vi "Interpolate Points.vi"(1 "End Point":cluster{"X":dbl, "Y":dbl}, 2 "Distance between Points":dbl, 3 "Start Point":cluster{"X":dbl, "Y":dbl}) -> (0 "Output Point Array":cluster{"X":dbl, "Y":dbl}[](array[cluster]))   [LabVIEW 2013]
doc: "This VI interpolates at specified intervals between two points."
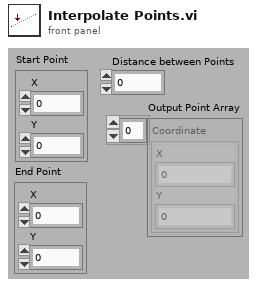
[diagram p1: front panel]
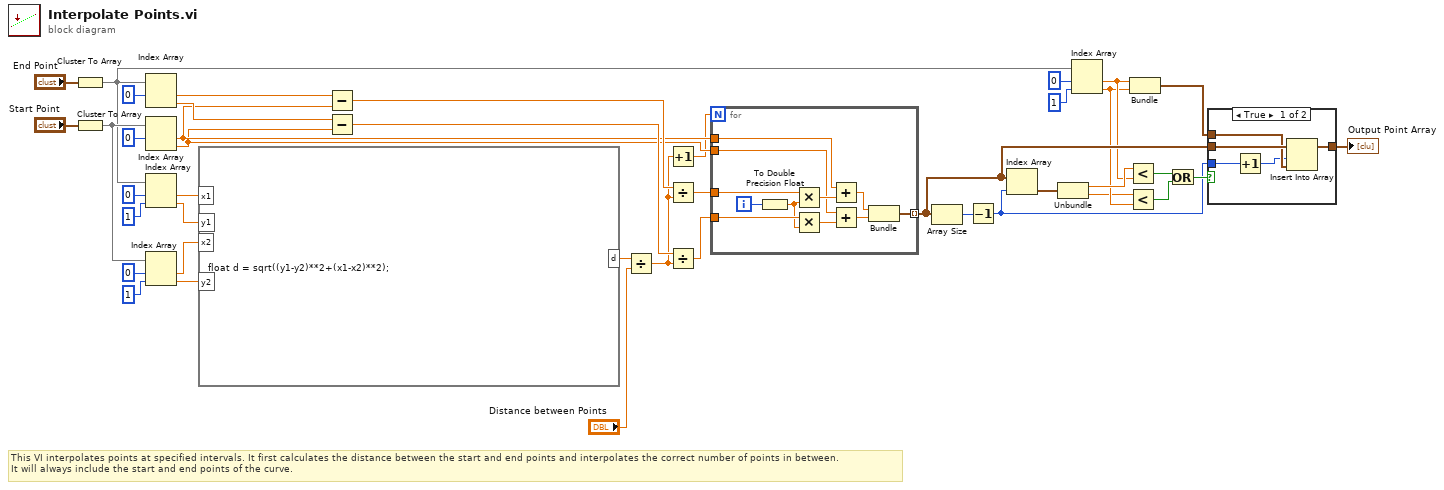
[diagram p0: block diagram]
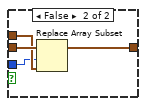
[diagram p2: hidden frame]
diagram:
  # "This VI interpolates points at specified intervals. It first calculates the distance between the start and end points and interpolates the correct number of points in between. \nIt will always include the start and end points of the curve."
  n1 = Cluster To Array(cluster="End Point") -> (array=w13:dbl[])
  n2 = Cluster To Array(cluster="Start Point") -> (array=w14:dbl[])
  n3 = Index Array(array=w13, index #1=0 ("index")) -> (element #1=w39:dbl, element #2=w36:dbl)  [unwired: 1 in]
  n4 = Index Array(array=w14, index #1=0 ("index")) -> (element #1=w35:dbl, element #2=w33:dbl)  [unwired: 1 in]
  n5 = Index Array(array=w13, index #1=0 ("index"), index #2=1 ("index")) -> (element #1=w24:dbl, element #2=w23:dbl)
  n6 = Index Array(array=w14, index #1=0 ("index"), index #2=1 ("index")) -> (element #1=w26:dbl, element #2=w25:dbl)
  n7 = formula code="float d = sqrt((y1-y2)**2+(x1-x2)**2);"("x1"=w24, "y1"=w23, "x2"=w26, "y2"=w25) -> ("d"=w22:dbl)
  n8 = Subtract(x=w39, y=w35) -> (x-y=w38:dbl)
  n9 = Subtract(x=w36, y=w33) -> (x-y=w37:dbl)
  n10 = Divide(x=w22, y="Distance between Points") -> (x/y=w20:dbl)
  n11 = Increment(x=w20) -> (x+1=w31:dbl)
  n12 = Divide(x=w38, y=w20) -> (x/y=w34:dbl)
  n13 = Divide(x=w37, y=w20) -> (x/y=w32:dbl)
  n14 = for {
    N: w31 -> [_]
    tunnel: w35 -> [w52]
    tunnel: w34 -> [w51]
    tunnel: w33 -> [w49]
    tunnel: w32 -> [w48]
    tunnel: [w44] -> w7 mode=indexing
    i -> [w43]
    n15 = To Double Precision Float(number=w43) -> (double precision float=w42:dbl)
    n16 = Multiply(x=w51, y=w42) -> (x*y=w50:dbl)
    n17 = Multiply(x=w48, y=w42) -> (x*y=w47:dbl)
    n18 = Add(x=w52, y=w50) -> (x+y=w46:dbl)
    n19 = Add(x=w49, y=w47) -> (x+y=w45:dbl)
    n20 = Bundle(w46, w45) -> (w44:cluster{dbl, dbl})  [unwired: 1 out]
  }
  n21 = Array Size(array=w7) -> (size(s)=w16:i32)
  n22 = Decrement(x=w16) -> (x-1=w6:i32)
  n23 = Index Array(array=w7, index=w6) -> (element=w5:cluster{dbl, dbl})
  n24 = Unbundle(w5) -> (w4:dbl, w1:dbl)
  n25 = Index Array(array=w13, index #1=0 ("index"), index #2=1 ("index")) -> (element #1=w3:dbl, element #2=w2:dbl)
  n26 = Less?(x=w4, y=w3) -> (x < y?=w9:bool)
  n27 = Less?(x=w1, y=w2) -> (x < y?=w10:bool)
  n28 = Bundle("X"=w3, "X"=w2) -> (w17:cluster{"X":dbl, "X":dbl})  [unwired: 1 in]
  n29 = Or(x=w9, y=w10) -> (x .or. y?=w8:bool)
  n30 = case shown="True" w8 {
    tunnel: w7 -> [w57 w61]
    tunnel: w17 -> [w56 w60]
    tunnel: w6 -> [w54 w59]
    tunnel: [w55 w58] -> w11
    frame True {
      n31 = Increment(x=w54) -> (x+1=w53:i32)
      n32 = Insert Into Array(array=w57, index=w53, new element=w56) -> (w55:cluster{dbl, dbl}[])
    }
    frame False {
      n33 = Replace Array Subset(array=w61, new element=w60, index=w59) -> (w58:cluster{dbl, dbl}[])
    }
  }
  "Output Point Array" <- w11
